vi "dl950_wave_20240517.vi"() -> ()   [LabVIEW 2019]
uses:
  84875dfb-7841-4e1b-95d2-ad8c7a5fa926.vi
  <vilib>/DAQmx/write.llb/DAQmx Write (Analog 1D Wfm NChan NSamp).vi
  <vilib>/DAQmx/create/channels.llb/DAQmx Create Channel (AO-Voltage-Basic).vi
  <vilib>/DAQmx/configure/timing.llb/DAQmx Timing (Sample Clock).vi
  <vilib>/DAQmx/miscellaneous.llb/DAQmx Fill In Error Info.vi
  <instrlib>/Yokogawa DL950 Series/Yokogawa DL950 Series.lvlib
  <resource>/objmgr/daqmx.rc
  <vilib>/measure/NI_MABase.lvlib
panel:
  in  "items":i32[](array[ring]) items=["Peak to Peak", "Amplitude", "Max", "Min", "High", "Low", "Average", "Middle", "Rms", "Standard Deviation", "+Overshoot", "-Overshoot", "Rise", "Fall", "Frequency", "Period", "+Width", "-Width", "Duty Cycle", "Pulse Count", "Burst1 Width", "Burst2 Width", "Average Frequency", "Average Period", "Int1TY", "Int2TY"]
  in  "enable":bool[](array[boolean])
  in  "stop 2":bool
  in  "Tab Control":enum32{"NI AO", "DL950", "load file"}(tab)
  in  "AO Stop":bool
  in  "AO Start":bool
  in  "Physical Channel(s)":tag="cDAQ1Mod1/ao0"
  in  "Min Voltage":dbl=-5.0
  in  "Max Voltage":dbl=5.0
  in  "Sample Clock Source":tag="OnboardClock"
  in  "Sample Rate":dbl=1000.0
  in  "Number of Samples":i32=100
  in  "Output Array":T1(array[cluster])=[{"Waveform Type"=2, "Amplitude"=1.0, "Frequency"=100.0}] {"Frequency" format="%0.2p"; "Amplitude" format="%0.2p"; "Waveform Type" items=["Sine Wave", "Triangle Wave", "Square Wave", "Sawtooth Wave"]}
  in  "offset":dbl=1.0 format="%#_13g"
  in  "square wave duty cycle (%)":dbl=50.0 format="%0.2f"
  out "Waveform Graph 2":waveform(dbl)[](graph)=[{"t0"=timestamp(0 s since 1904-01-01), "dt"=0.001, "Y"=[]}]
  in  "Sample Mode":i32(ring)=10178 items=["Finite Samples", "Continuous Samples", "Hardware Timed Single Point"]
  in  "DAQ Simulation":bool
  out "data":T2
  out "Name of Items":string[](array[string])
  out "Items":dbl[](array[numeric])
  in  "Item Measure":bool
  in  "Item Measure":bool
  in  "Set Apply":bool
  in  "Normal":bool
  in  "open":dbl
  in  "short":dbl
  in  "Open":bool
  in  "Short":bool
  out "Waveform Graph":waveform(dbl)(graph)
  in  "Timeout (10000 ms)":u32=10000
  in  "Sub Channel (0: None)":i16(ring) items=["None", "SCH1", "SCH2", "SCH3", "SCH4", "SCH5", "SCH6", "SCH7", "SCH8", "SCH9", "SCH10", "SCH11", "SCH12", "SCH13", "SCH14", "SCH15", "SCH16", "SCH17", "SCH18", "SCH19", "SCH20", "SCH21", "SCH22", "SCH23", "SCH24", "SCH25", "SCH26", "SCH27", "SCH28", "SCH29", "SCH30", "SCH31", "SCH32", "SCH33", "SCH34", "SCH35", "SCH36", "SCH37", "SCH38", "SCH39", "SCH40", "SCH41", "SCH42", "SCH43", "SCH44", "SCH45", "SCH46", "SCH47", "SCH48", "SCH49", "SCH50", "SCH51", "SCH52", "SCH53", "SCH54", "SCH55", "SCH56", "SCH57", "SCH58", "SCH59", "SCH60", "SCH61", "SCH62", "SCH63", "SCH64"]
  in  "Source (1: CH1)":u16(ring)=1 items=["", "CH1", "CH2", "CH3", "CH4", "CH5", "CH6", "CH7", "CH8", "CH9", "CH10", "CH11", "CH12", "CH13", "CH14", "CH15", "CH16", "MATH1", "MATH2", "MATH3", "MATH4", "MATH5", "MATH6", "MATH7", "MATH8", "EVENT"]
  in  "VISA resource name":refnum<visa-resource-name>="TCPIP0::192.168.0.100::inst0::INSTR"
  in  "Connect":bool
  in  "disconnect":bool
  in  "start":bool
  in  "stop":bool
  in  "freerun":bool
  in  "aquisition":bool
  in  "String":string=":TRIG:SOUT:TYPE ACQ;"
  in  "aquisition STOP":bool
  in  "Vertical Coupling (1: DC)":i32(ring)=1 items=["AC", "DC", "Ground", "AC-RMS", "DC-RMS"]
  in  "Vertical Division (20: 50)":i32(ring)=20 items=["0.1m", "0.2m", "0.5m", "1m", "2m", "5m", "10m", "20m", "50m", "100m", "200m", "500m", "1", "2", "4", "5", "8", "10", "20", "40", "50", "80", "100", "200", "400", "500", "800", "1k", "2k", "4k", "5k", "8k", "10k", "20k", "25k", "50k", "100k", "250k", "500k", "1000k"]
  in  "Time Division (12: 1ms)":i32(ring)=12 items=["100ns", "200ns", "500ns", "1us", "2us", "5us", "10us", "20us", "50us", "100us", "200us", "500us", "1ms", "2ms", "5ms", "10ms", "20ms", "50ms", "100ms", "200ms", "500ms", "1s", "2s", "3s", "4s", "5s", "6s", "10s", "20s", "30s", "1min", "2min", "3min", "4min", "5min", "6min", "10min", "12min", "30min", "1hour", "2hour", "3hour", "4hour", "5hour", "6hour", "8hour", "10hour", "12hour", "1day", "2day", "3day", "4day", "5day"]
  out "Array":dbl[](array[numeric])
  in  "Record Length (0: 10k)":i32(ring) items=["10k", "25k", "50k", "100k", "250k", "500k", "1M", "2.5M", "5M", "10M", "25M", "50M", "100M", "250M", "500M", "1G", "2G", "4G", "5G", "10G", "20G", "50G"]
  in  "Acquisition Mode (0: Normal)":i32(ring) items=["Normal", "Average", "Envelope"]
  in  "inpuPara":T3={"Rising[%] 1"=63.0, "Rising[%] 2"=99.0, "Falling[%]"=37.0}
  out "calculation":u32
  out "itemMeasure":u32
  out "Oscilloscope":u32
  out "Loop":u32
  in  "End Point(1000)":i64=1000
  in  "Record Number (0)":i32
  in  "Start Point(0)":i64
  out "task out":refnum<k21>
  out "SampQuant.SampPerChan":dbl
  out "SampClk.Rate":dbl
  in  "Channel (1: CH1)":u16(ring)=1 items=["", "CH1", "CH2", "CH3", "CH4", "CH5", "CH6", "CH7", "CH8", "CH9", "CH10", "CH11", "CH12", "CH13", "CH14", "CH15", "CH16", "RMATH1", "RMATH2", "RMATH3", "RMATH4", "RMATH5", "RMATH6", "RMATH7", "RMATH8", "RMATH9", "RMATH10", "RMATH11", "RMATH12", "RMATH13", "RMATH14", "RMATH15", "RMATH16"]
  in  "sub Channel (1: CH1)":u16(ring)=1 items=["", "CH1", "CH2", "CH3", "CH4", "CH5", "CH6", "CH7", "CH8", "CH9", "CH10", "CH11", "CH12", "CH13", "CH14", "CH15", "CH16", "RMATH1", "RMATH2", "RMATH3", "RMATH4", "RMATH5", "RMATH6", "RMATH7", "RMATH8", "RMATH9", "RMATH10", "RMATH11", "RMATH12", "RMATH13", "RMATH14", "RMATH15", "RMATH16"]
  in  "Enable Channel (True)":bool=TRUE
  in  "Reset":bool
  in  "write":bool
  out "read buffer":string
  in  "String 2":string=":FILE:SAVE?;"
  in  "Numeric":u32=20
  in  "response":bool
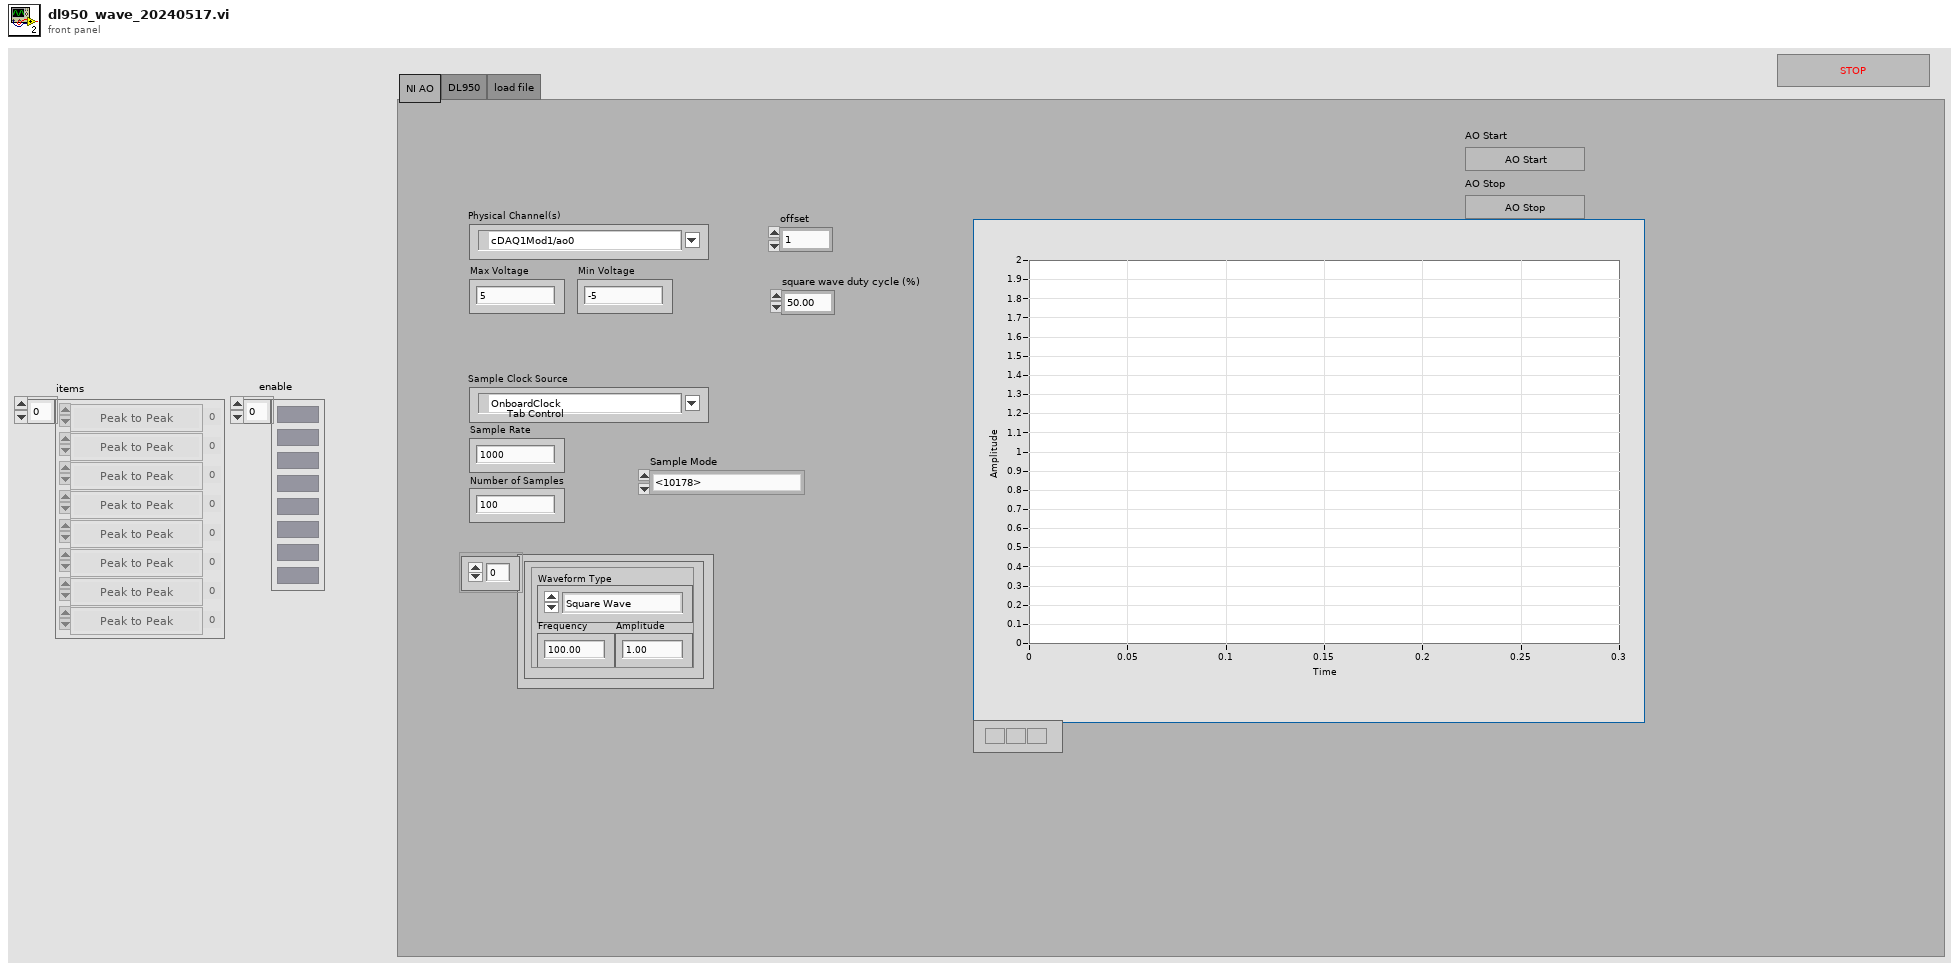
[diagram p1: front panel]
types:
  T1 = cluster{"Waveform Type":u16, "Amplitude":dbl, "Frequency":dbl}[]
  T2 = cluster{"pulse":i32, "Rising[%] 1":dbl, "Rising[%] 2":dbl, "Falling[%]":dbl, "R_max":dbl}
  T3 = cluster{"Rising[%] 1":dbl, "Rising[%] 2":dbl, "Falling[%]":dbl}
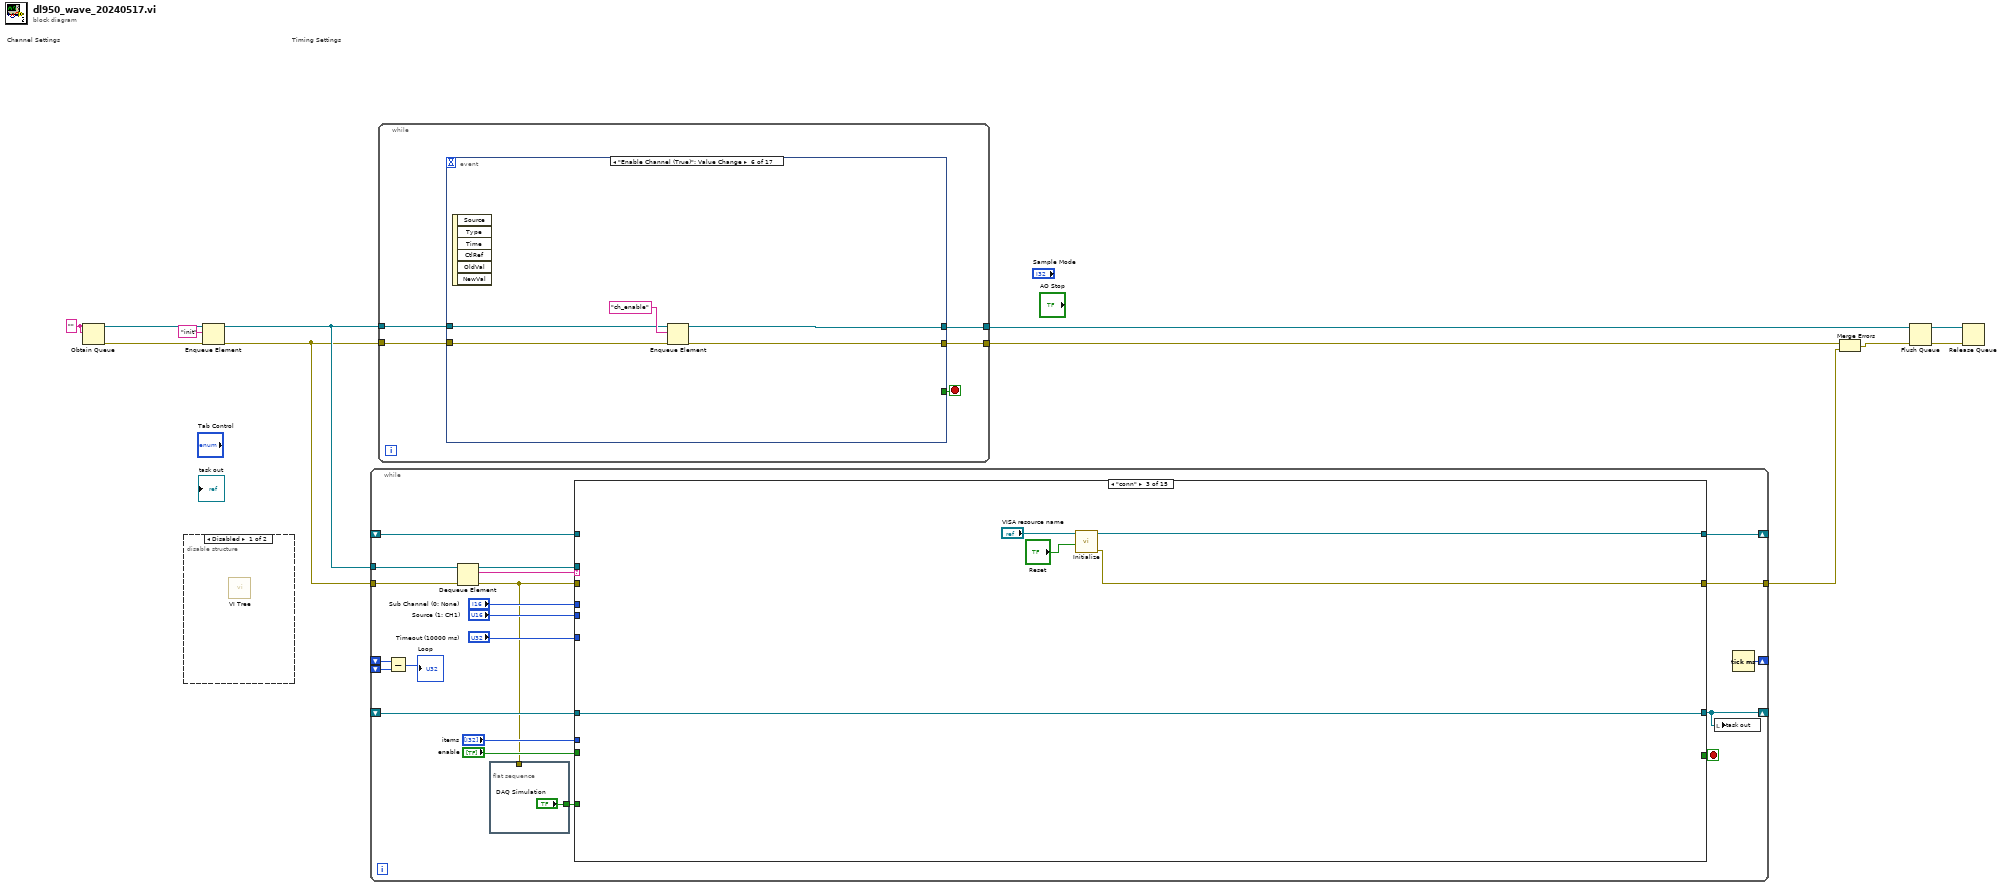
[diagram p0: block diagram]
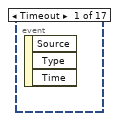
[diagram p3: hidden frame]
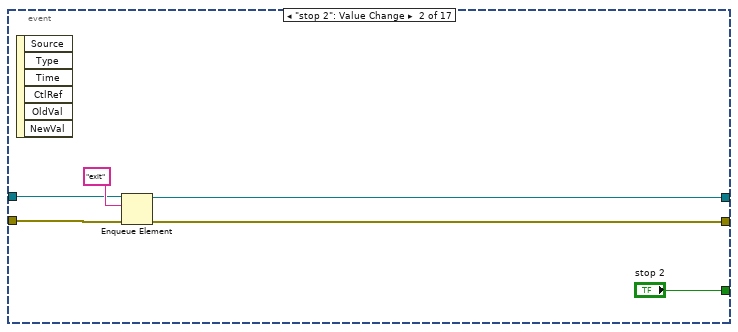
[diagram p4: hidden frame]
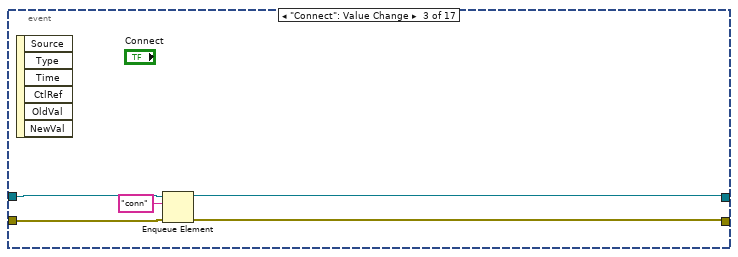
[diagram p5: hidden frame]
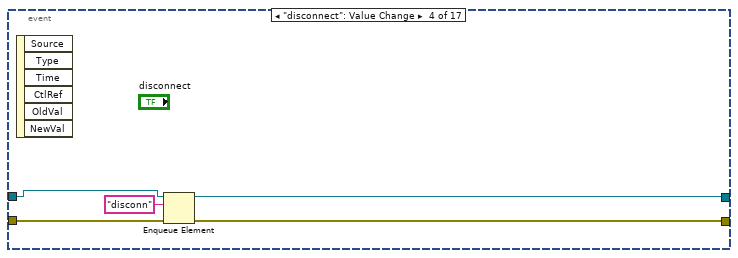
[diagram p6: hidden frame]
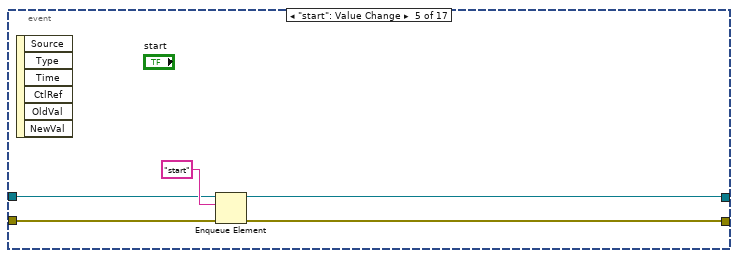
[diagram p7: hidden frame]
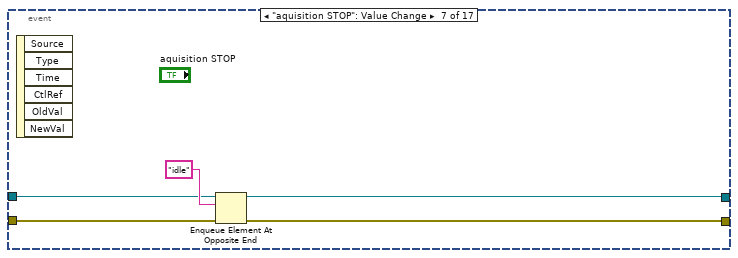
[diagram p8: hidden frame]
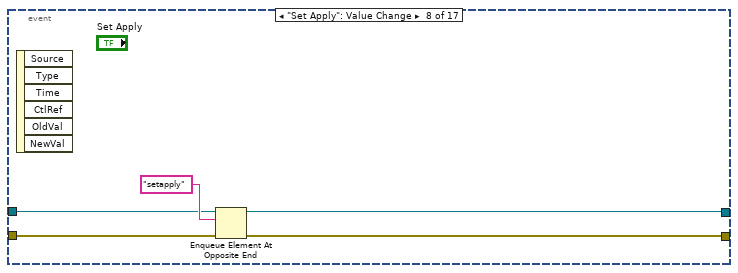
[diagram p9: hidden frame]
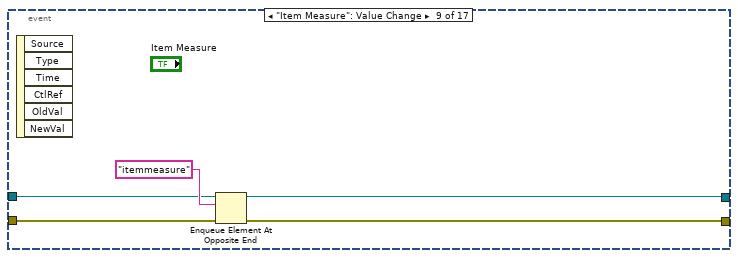
[diagram p10: hidden frame]
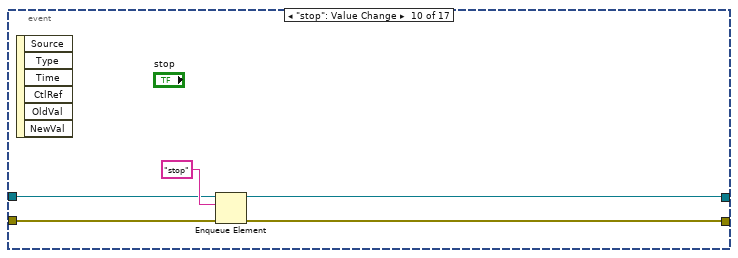
[diagram p11: hidden frame]
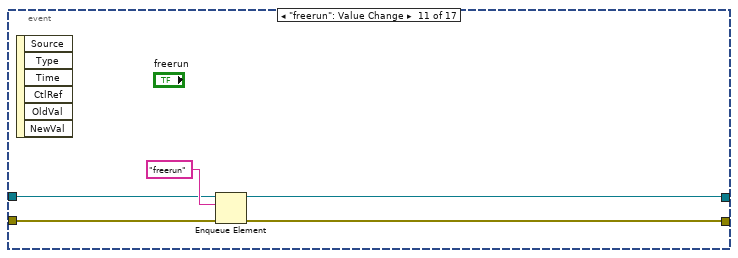
[diagram p12: hidden frame]
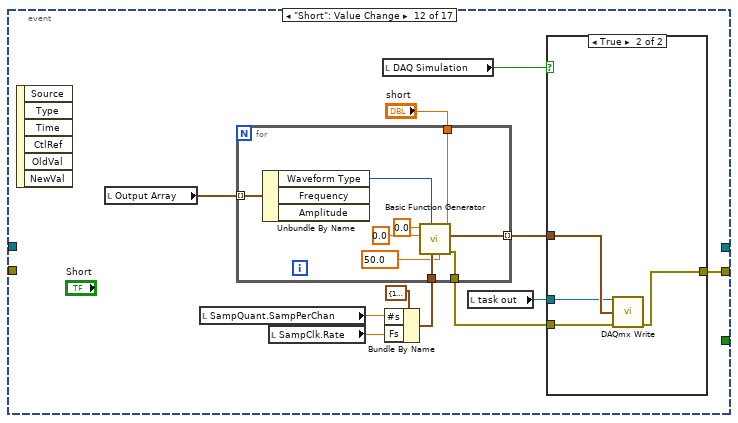
[diagram p13: hidden frame]
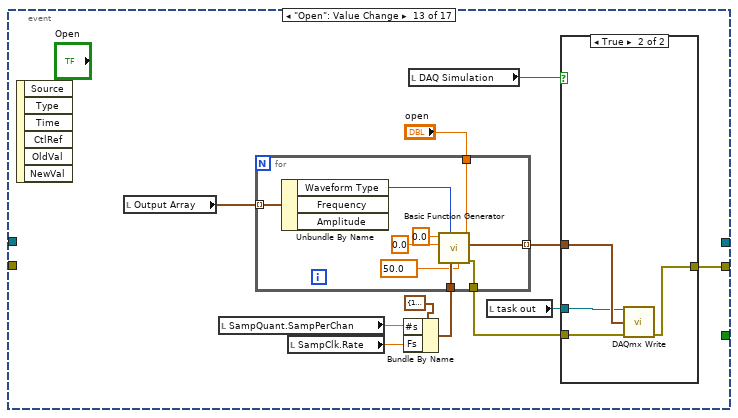
[diagram p15: hidden frame]
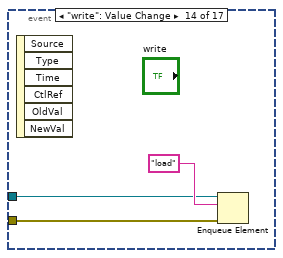
[diagram p17: hidden frame]
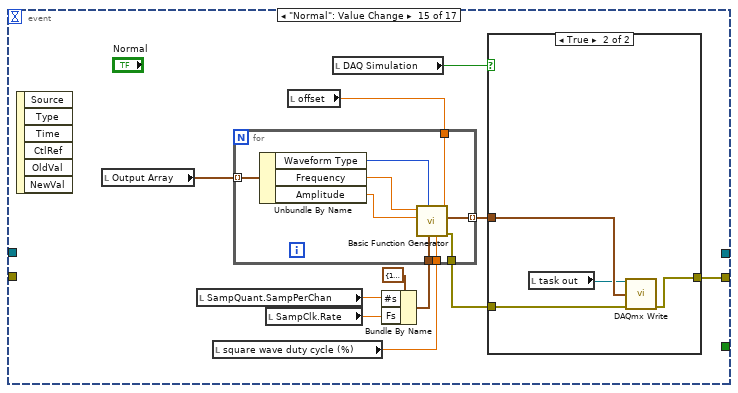
[diagram p18: hidden frame]
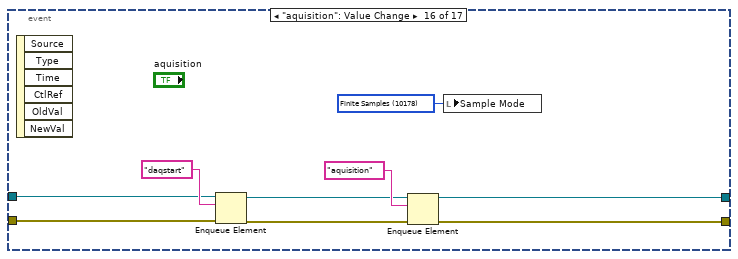
[diagram p20: hidden frame]
diagram:
  w1 = "" ("name (unnamed)")
  # "Timing Settings"
  # "Channel Settings"
  n1 = Obtain Queue(name (unnamed)=w1, element data type=w1) -> (queue out=w12:refnum<queue>, error out=w11:errorcluster)  [unwired: 3 in, 1 out]
  n2 = disable-structure shown="Disabled" {
    frame Disabled {
      n3 = call <instrlib>:"VI Tree.vi"() -> ()  [unwired: 12 in]
    }
    frame Enabled {
    }
  }
  n4 = Enqueue Element(queue=w12, element="init", error in (no error)=w11) -> (queue out=w9:refnum<queue>, error out=w8:errorcluster)  [unwired: 1 in, 1 out]
  n5 = while {
    tunnel: w9 -> [w33]
    tunnel: w8 -> [w32]
    tunnel: [w29] -> w6
    shift-right: [w28] -> _
    shift-left: _ -> [w27]
    shift-right: [w22] -> _
    shift-left: _ -> [w21]
    shift-left: _ -> [w20]
    shift-right: [w17] -> _
    shift-left: _ -> [w18]
    stop <- w30 stop-if-true
    n6 = Subtract(x=w21, y=w20) -> (x-y=→"Loop":u32)
    n7 = Dequeue Element(queue=w33, error in (no error)=w32) -> (queue out=w23:refnum<queue>, element=w31:string, error out=w14:errorcluster)  [unwired: 1 in, 1 out]
    n8 = flat-sequence {
      tunnel: w14 -> [_]
      tunnel: ["DAQ Simulation"] -> w13
      frame #0 {
      }
    }
    n9 = case shown="\"conn\"" w31 {
      tunnel: [_ TRUE _ _ _ _ _ _ _ _ _ _ _ _ _] -> w30
      tunnel: [w36 w40 w42 w50 w80 w96 w99 w106 w112 w122 w210 w238 w284 w295 w301] -> w29
      tunnel: w14 -> [w36 w40 _ w52 w64 w97 w100 w107 w113 w148 w211 _ w290 w296 w302]
      tunnel: [w37 w39 w43 w51 w81 w95 w101 w108 w114 w134 w212 w239 w292 w298 w305] -> w28
      tunnel: w27 -> [w37 w39 _ w53 w65 w95 w102 w109 w115 w146 w213 w239 w292 w298 w305]
      tunnel: "Source (1: CH1)" -> [_ _ _ _ w63 _ _ _ _ w132 w207 _ _ _ _]
      tunnel: "Sub Channel (0: None)" -> [_ _ _ _ w79 _ _ _ _ w131 w206 _ _ _ _]
      tunnel: "Timeout (10000 ms)" -> [_ _ _ _ _ _ _ _ _ w153 _ _ _ _ _]
      tunnel: w23 -> [_ _ _ _ _ _ _ _ _ w149 _ _ w289 w297 _]
      tunnel: [w35 w38 w45 w54 w83 w94 w98 w104 w110 w140 w214 w237 w285 w294 w307] -> w17
      tunnel: w18 -> [w35 w38 w45 w54 w83 w94 w98 w104 w110 w141 w214 _ w286 w294 w307]
      tunnel: "items" -> [_ _ _ _ w78 _ _ _ _ w130 w209 _ _ _ _]
      tunnel: "enable" -> [_ _ _ _ w77 _ _ _ _ w129 w208 _ _ _ _]
      tunnel: w13 -> [_ _ _ _ _ _ _ _ _ w116 _ w236 _ w293 _]
      frame "False", Default {
      }
      frame "exit" {
      }
      frame "conn" {
        n10 = call <instrlib>:"Initialize.vi"("Reset (True)"="Reset", "VISA resource name"="VISA resource name") -> ("error out"=w42:errorcluster, "VISA resource name out"=w43:refnum<visa-resource-name>)  [unwired: 8 in]
      }
      frame "ch_enable" {
        n11 = call <instrlib>:"Configure Channel.vi"("VISA resource name"=w53, "Channel (1: CH1)"="Channel (1: CH1)", "Enable Channel (True)"="Enable Channel (True)", "sub Channel (1: CH1)"="sub Channel (1: CH1)", "error in (no error)"=w52) -> ("VISA resource name out"=w51:refnum<visa-resource-name>, "error out"=w50:errorcluster)  [unwired: 9 in]
      }
      frame "setapply" {
        n12 = Format Into String ("文字列にフォーマット")(format string="CHAN%d:", w63) -> (resulting string=w72:string)  [unwired: 2 in, 1 out]
        n13 = Pick Line ("ライン選択")(string ("")=w72, multi-line string="COUP AC;\nCOUP DC;\nCOUP GND;\nCOUP ACRMS;\nCOUP DCRMS;", line index="Vertical Coupling (1: DC)") -> (output string=w73:string)
        n14 = call <instrlib>:"Configure Acquisition.vi"("VISA resource name"=w65, "Record Length (0: 10k)"="Record Length (0: 10k)", "Acquisition Mode (0: Normal)"="Acquisition Mode (0: Normal)", "error in (no error)"=w64) -> ("VISA resource name out"=w60:refnum<visa-resource-name>, "error out"=w58:errorcluster)  [unwired: 10 in]
        n15 = call <instrlib>:"Configure Timebase.vi"("VISA resource name"=w60, "Time Division (12: 1ms)"="Time Division (12: 1ms)", "error in (no error)"=w58) -> ("VISA resource name out"=w59:refnum<visa-resource-name>, "error out"=w57:errorcluster)  [unwired: 11 in]
        n16 = Pick Line ("ライン選択")(string ("")=w73, multi-line string="VDIV 0.0001;\nVDIV 0.0002;\nVDIV 0.0005;\nVDIV 0.001;\nVDIV 0.002;\nVDIV 0.005;\nVDIV 0.01;\nVDIV 0.02;\nVDIV 0.05;\nVDIV 0.1;\nVDIV 0.2;\nVDIV 0.5;\nVDIV 1;\nVDIV 2;\nVDIV 4;\nVDIV 5;\nVDIV 8;\nVDIV 10;\nVDIV 20;\nVDIV 40;\nVDIV 50;\nVDIV 80;\nVDIV 100;\nVDIV 200;\nVDIV 400;\nVDIV 500;\nVDIV 800;\nVDIV 1000;\nVDIV 2000;\nVDIV 4000;\nVDIV 5000;\nVDIV 8000;\nVDIV 10000;\nVDIV 20000;\nVDIV 25000;\nVDIV 50000;\nVDIV 100000;\nVDIV 250000;\nVDIV 500000;\nVDIV 1000000;", line index="Vertical Division (20: 50)") -> (output string=w68:string)
        n17 = VISA Write ("VISA書き込み")(VISA resource name=w59, write buffer=w68, error in (no error)=w57) -> (VISA resource name out=w56:refnum<visa-resource-name>, error out=w55:errorcluster)  [unwired: 1 out]
        n18 = property on="Measurement Item (0: Peak to Peak)" class="Ring (strict)"(error in=w55) -> (error out=w76:errorcluster, "Strings []"=w75:string[])  [unwired: 1 in, 1 out]
        n19 = for {
          tunnel: w79 -> [w85]
          tunnel: w63 -> [w84]
          shift-right: [w92] -> w81
          shift-left: w56 -> [w93]
          shift-right: [w90] -> w80
          shift-left: w76 -> [w91]
          tunnel: w77 -> [w86] mode=indexing
          tunnel: w78 -> [w88] mode=indexing
          tunnel: w75 -> [w89]
          tunnel: [w87] -> w74 mode=indexing if=w86
          n20 = call <instrlib>:"Configure Measurement Item.vi"("VISA resource name"=w93, "Source (1: CH1)"=w84, "Sub Channel (0: None)"=w85, "Measurement Item (0: Peak to Peak)"=w88, "Enable Measurement Item (False)"=w86, "error in (no error)"=w91) -> ("VISA resource name out"=w92:refnum<visa-resource-name>, "error out"=w90:errorcluster)  [unwired: 8 in]
          n21 = Index Array(array=w89, index=w88) -> (element=w87:string)
        }
        "Name of Items" <- w74
      }
      frame "disconn" {
        n22 = call <instrlib>:"Close.vi"("error in (no error)"=w97, "VISA resource name"=w95) -> ("error out"=w96:errorcluster)  [unwired: 9 in]
      }
      frame "start" {
        w103 = ":STAR;"  # Initiate
        n23 = VISA Write ("VISA書き込み")(VISA resource name=w102, write buffer=w103, error in (no error)=w100) -> (VISA resource name out=w101:refnum<visa-resource-name>, error out=w99:errorcluster)  [unwired: 1 out]
      }
      frame "stop" {
        n24 = VISA Write ("VISA書き込み")(VISA resource name=w109, write buffer=":STOP;", error in (no error)=w107) -> (VISA resource name out=w108:refnum<visa-resource-name>, error out=w106:errorcluster)  [unwired: 1 out]
      }
      frame "freerun" {
        n25 = VISA Write ("VISA書き込み")(VISA resource name=w115, write buffer="String", error in (no error)=w113) -> (VISA resource name out=w114:refnum<visa-resource-name>, error out=w112:errorcluster)  [unwired: 1 out]
      }
      frame "aquisition" {
        w147 = ":STAR;"  # Initiate
        n26 = Enqueue Element(queue=w149, element="aquisition", error in (no error)=w148) -> (error out=w145:errorcluster)  [unwired: 1 in, 2 out]
        n27 = VISA Write ("VISA書き込み")(VISA resource name=w146, write buffer=w147, error in (no error)=w145) -> (VISA resource name out=w143:refnum<visa-resource-name>, error out=w139:errorcluster)  [unwired: 1 out]
        n28 = call "Stall Data Flow.vim"("value in"=w139, "milliseconds to wait"=u32 200) -> ("value out"=w137:errorcluster)  [unwired: 1 out]
        n29 = case shown="True" w116 {
          tunnel: w141 -> [w156 w160]
          tunnel: [w156 w159] -> w140
          tunnel: w137 -> [w155 w158]
          tunnel: [w155 w157] -> w136
          frame False {
          }
          frame True {
            n30 = call <vilib>:"DAQmx Start Task.vi"("task/channels in"=w160, "error in"=w158) -> ("task out"=w163:refnum<k21>, "error out"=w162:errorcluster)  [unwired: 12 in]
            n31 = call <vilib>:"DAQmx Wait Until Done.vi"("task/channels in"=w163, "error in"=w162) -> ("task out"=w161:refnum<k21>, "error out"=w157:errorcluster)  [unwired: 12 in]
            n32 = call <vilib>:"DAQmx Stop Task.vi"("task/channels in"=w161, "error in"=w157) -> ("task out"=w159:refnum<k21>)  [unwired: 12 in, 1 out]
          }
        }
        n33 = VISA Write ("VISA書き込み")(VISA resource name=w143, write buffer=":STOP;", error in (no error)=w136) -> (VISA resource name out=w142:refnum<visa-resource-name>, error out=w121:errorcluster)  [unwired: 1 out]
        n34 = flat-sequence {
          tunnel: w121 -> [w165]
          tunnel: [w165] -> w120
          tunnel: [w164] -> w117
          frame #0 {
            n35 = Tick Count (ms)() -> (millisecond timer value=w164:u32)
          }
        }
        n36 = call "waveAquis.vi"("Timeout (10000 ms)"=w153, "Sub Channel(0: None)"=w131, "End Point(1000)"=i64 -1, "Source (1: CH1)"=w132, "error in (no error)"=w120, "Start Point(0)"="Start Point(0)", "Record Number (0)"="Record Number (0)", "VISA resource name"=w142) -> ("error out"=w125:errorcluster, "Waveform Data"=w128:waveform(dbl), "VISA resource name out"=w135:refnum<visa-resource-name>)  [unwired: 1 in]
        "Waveform Graph" <- w128
        n37 = flat-sequence {
          tunnel: w125 -> [w173]
          tunnel: [w173] -> w124
          tunnel: [w172] -> w118
          frame #0 {
            n38 = Tick Count (ms)() -> (millisecond timer value=w172:u32)
          }
        }
        n39 = case shown="True" "Item Measure" {
          tunnel: w135 -> [w175 w184]
          tunnel: [w175 w183] -> w134
          tunnel: w125 -> [w174 w182]
          tunnel: [w174 w181] -> w122
          tunnel: w132 -> [_ w180]
          tunnel: w131 -> [_ w179]
          tunnel: w130 -> [_ w178]
          tunnel: w129 -> [_ w177]
          frame False {
          }
          frame True {
            n40 = for {
              tunnel: w184 -> [w193]
              tunnel: [w192] -> w183
              tunnel: w182 -> [w191]
              tunnel: [w190] -> w181
              tunnel: w178 -> [w189] mode=indexing
              tunnel: w177 -> [w188] mode=indexing
              tunnel: w180 -> [w187]
              tunnel: w179 -> [w186]
              tunnel: [w185] -> w176 mode=indexing
              n41 = case shown="True" w188 {
                tunnel: w193 -> [w196 w204]
                tunnel: [w196 w203] -> w192
                tunnel: w191 -> [w195 w202]
                tunnel: [w195 w201] -> w190
                tunnel: w189 -> [_ w200]
                tunnel: w187 -> [_ w199]
                tunnel: w186 -> [_ w198]
                tunnel: [0.0 ("Measurement Value") w197] -> w185
                frame False {
                }
                frame True {
                  n42 = call <instrlib>:"Read Waveform Measurement.vi"("VISA resource name"=w204, "Source (1: CH1)"=w199, "Sub Channel (0: None)"=w198, "Measurement Item (0: Peak to Peak)"=w200, "error in (no error)"=w202) -> ("VISA resource name out"=w203:refnum<visa-resource-name>, "Measurement Value"=w197:dbl, "error out"=w201:errorcluster)  [unwired: 8 in]
                }
              }
            }
            "Items" <- w176
          }
        }
        n43 = Subtract(x=w118, y=w117) -> (x-y=→"Oscilloscope":u32)
        n44 = call "signalAnalysis.vi"("error in (no error)"=w124, "inpuPara"="inpuPara", "data_scope"=w128) -> ("error out"=w123:errorcluster, "data"=→"data":T2)  [unwired: 7 in]
        n45 = flat-sequence {
          tunnel: w123 -> [_]
          tunnel: w118 -> [w170]
          frame #0 {
            n46 = Tick Count (ms)() -> (millisecond timer value=w171:u32)
            n47 = Subtract(x=w171, y=w170) -> (x-y=→"calculation":u32)
          }
        }
        n48 = flat-sequence {
          tunnel: w118 -> [w167]
          tunnel: w122 -> [_]
          frame #0 {
            n49 = Tick Count (ms)() -> (millisecond timer value=w168:u32)
            n50 = Subtract(x=w168, y=w167) -> (x-y=→"itemMeasure":u32)
          }
        }
      }
      frame "itemmeasure" {
        n51 = for {
          tunnel: w213 -> [w223]
          tunnel: [w222] -> w212
          tunnel: w211 -> [w221]
          tunnel: [w220] -> w210
          tunnel: w209 -> [w219] mode=indexing
          tunnel: w208 -> [w218] mode=indexing
          tunnel: w207 -> [w217]
          tunnel: w206 -> [w216]
          tunnel: [w215] -> w205 mode=indexing
          n52 = case shown="True" w218 {
            tunnel: w223 -> [w226 w234]
            tunnel: [w226 w233] -> w222
            tunnel: w221 -> [w225 w232]
            tunnel: [w225 w231] -> w220
            tunnel: w219 -> [_ w230]
            tunnel: w217 -> [_ w229]
            tunnel: w216 -> [_ w228]
            tunnel: [0.0 ("Measurement Value") w227] -> w215
            frame False {
            }
            frame True {
              n53 = call <instrlib>:"Read Waveform Measurement.vi"("VISA resource name"=w234, "Source (1: CH1)"=w229, "Sub Channel (0: None)"=w228, "Measurement Item (0: Peak to Peak)"=w230, "error in (no error)"=w232) -> ("VISA resource name out"=w233:refnum<visa-resource-name>, "Measurement Value"=w227:dbl, "error out"=w231:errorcluster)  [unwired: 8 in]
            }
          }
        }
        "Array" <- w205
      }
      frame "daqstart" {
        n54 = local read "Sample Mode"() -> (w235:i32)
        n55 = case shown="True" w236 {
          tunnel: [_ w243] -> w238
          tunnel: [refnum<k21> refnum ("task out") w242] -> w237
          tunnel: w235 -> [_ w241]
          frame False {
          }
          frame True {
            n56 = stacked-sequence {
              seq-local: [w247 _] -> [_ w265]
              seq-local: [w246 _] -> [_ w263]
              seq-local: [w245 _] -> [_ w264]
              tunnel: [w246 _] -> _
              tunnel: [w245 _] -> _
              tunnel: [w247 _] -> _
              tunnel: [w248 _] -> w243
              tunnel: [_ w261] -> w242
              tunnel: w241 -> [w244 w262]
              frame #0 {
                n57 = call-poly <vilib>:"DAQmx Create Virtual Channel.vi"("maximum value"="Max Voltage", "minimum value"="Min Voltage", "physical channels"="Physical Channel(s)") -> ("task out"=w255:refnum<k21>, "error out"=w256:errorcluster)  [unwired: 11 in]
                n58 = call-poly <vilib>:"DAQmx Timing.vi"("task/channels in"=w255, "sample mode"=w244, "samples per channel"="Number of Samples", "rate"="Sample Rate", "source"="Sample Clock Source", "error in"=w256) -> ("task out"=w258:refnum<k21>, "error out"=w257:errorcluster)  [unwired: 8 in]
                n59 = property class="DAQmx Timing"(reference=w258, error in=w257) -> (reference out=w247:refnum<k21>, error out=w248:errorcluster, "SampQuant.SampPerChan"=w246:dbl, "SampClk.Rate"=w245:dbl)
                "SampQuant.SampPerChan" <- w246
                "SampClk.Rate" <- w245
              }
              frame #1 {
                n60 = Bundle By Name(cluster=cluster{"Fs":dbl, "#s":dbl} {"Fs"=1000.0, "#s"=1000.0} ("sampling info"), "#s"=w263, "Fs"=w264) -> (w267:cluster{"Fs":dbl, "#s":dbl})
                n61 = for {
                  tunnel: w267 -> [w283]
                  tunnel: [w282] -> w268
                  tunnel: "Output Array" -> [w281] mode=indexing
                  tunnel: [w277] -> w270 mode=indexing
                  n62 = Unbundle By Name(w281) -> ("Waveform Type"=w280:u16, "Frequency"=w279:dbl, "Amplitude"=w278:dbl)
                  n63 = call <vilib>:"Basic Function Generator.vi"("offset"="offset", "square wave duty cycle (%)"="square wave duty cycle (%)", "sampling info"=w283, "signal type"=w280, "amplitude"=w278, "frequency"=w279) -> ("error out"=w282:errorcluster, "signal out"=w277:waveform(dbl))  [unwired: 3 in, 1 out]
                }
                "Waveform Graph 2" <- w270
                n64 = call-poly <vilib>:"DAQmx Write.vi"("task/channels in"=w265, "data"=w270, "error in"=w268) -> ("task out"=w260:refnum<k21>, "error out"=w259:errorcluster)  [unwired: 10 in, 1 out]
                n65 = case shown="1" w262 {
                  tunnel: [w271 w273] -> w261
                  tunnel: w260 -> [w271 w274]
                  tunnel: w259 -> [_ w272]
                  frame 0, Default {
                  }
                  frame 1 {
                    n66 = call <vilib>:"DAQmx Start Task.vi"("task/channels in"=w274, "error in"=w272) -> ("task out"=w273:refnum<k21>)  [unwired: 12 in, 1 out]
                  }
                }
              }
            }
          }
        }
      }
      frame "aostart" {
        n67 = Enqueue Element(queue=w289, element="aostart", error in (no error)=w290) -> (error out=w287:errorcluster)  [unwired: 1 in, 2 out]
        n68 = call <vilib>:"DAQmx Is Task Done.vi"("task/channels in"=w286, "error in"=w287) -> ("task out"=w285:refnum<k21>, "error out"=w284:errorcluster)  [unwired: 11 in, 1 out]
        n69 = Wait Until Next ms Multiple(millisecond multiple=u32 100) -> ()  [unwired: 1 out]
      }
      frame "idle" {
        n70 = Flush Queue(queue=w297, error in (no error)=w296) -> (error out=w295:errorcluster)  [unwired: 2 out]
        n71 = case shown="True" w293 {
          tunnel: w294 -> [_ w299]
          frame False {
          }
          frame True {
            n72 = call <vilib>:"DAQmx Clear Task.vi"("task in"=w299) -> ()  [unwired: 14 in, 1 out]
          }
        }
      }
      frame "load" {
        n73 = VISA Write ("VISA書き込み")(VISA resource name=w305, write buffer="String 2", error in (no error)=w302) -> (VISA resource name out=w304:refnum<visa-resource-name>, error out=w303:errorcluster)  [unwired: 1 out]
        n74 = case shown="True" "response" {
          tunnel: w304 -> [_ w312]
          tunnel: w303 -> [w308 w311]
          tunnel: [w308 w310] -> w301
          frame False {
          }
          frame True {
            n75 = VISA Read ("VISA読み取り")(VISA resource name=w312, byte count="Numeric", error in (no error)=w311) -> (read buffer=→"read buffer":string, error out=w310:errorcluster)  [unwired: 2 out]
          }
        }
      }
    }
    n76 = local write "task out"(w17) -> ()
    n77 = Tick Count (ms)() -> (millisecond timer value=w22:u32)
  }
  n78 = while {
    tunnel: w9 -> [w317]
    tunnel: w8 -> [w316]
    tunnel: [w315] -> w5
    tunnel: [w314] -> w7
    stop <- w318 stop-if-true
    n79 = event shown="[5] \"Enable Channel (True)\": Value Change" {
      selector: _ -> [_ _ _ _ _ _ _ _ _ _ _ _ _ _ _ _ _]
      dyn-events: _ -> [_ _ _ _ _ _ _ _ _ _ _ _ _ _ _ _ _]
      timeout: _ -> [_ _ _ _ _ _ _ _ _ _ _ _ _ _ _ _ _]
      tunnel: [_ "stop 2" _ _ _ _ _ _ _ _ _ _ _ _ _ _ _] -> w318
      tunnel: w317 -> [_ w322 w328 w333 w338 w343 w348 w353 w358 w363 w368 _ _ w421 _ w455 w461]
      tunnel: w316 -> [_ w321 w326 w332 w337 w341 w347 w352 w357 w362 w367 _ _ w420 _ w454 w459]
      tunnel: [_ w320 w327 w331 w336 w342 w346 w351 w356 w361 w366 _ _ _ _ w450 w464] -> w315
      tunnel: [_ w319 w325 w330 w335 w340 w345 w350 w355 w360 w365 w371 w397 _ w424 w449 w463] -> w314
      event Timeout {
        n80 = event-data() -> ()  [unwired: 1 in, 3 out]
      }
      event "stop 2": Value Change {
        n81 = event-data() -> ()  [unwired: 1 in, 6 out]
        n82 = Enqueue Element(queue=w322, element="exit", error in (no error)=w321) -> (queue out=w320:refnum<queue>, error out=w319:errorcluster)  [unwired: 1 in, 1 out]
      }
      event "Connect": Value Change {
        n83 = event-data() -> ()  [unwired: 1 in, 6 out]
        n84 = Enqueue Element(queue=w328, element="conn", error in (no error)=w326) -> (queue out=w327:refnum<queue>, error out=w325:errorcluster)  [unwired: 1 in, 1 out]
      }
      event "disconnect": Value Change {
        n85 = event-data() -> ()  [unwired: 1 in, 6 out]
        n86 = Enqueue Element(queue=w333, element="disconn", error in (no error)=w332) -> (queue out=w331:refnum<queue>, error out=w330:errorcluster)  [unwired: 1 in, 1 out]
      }
      event "start": Value Change {
        n87 = event-data() -> ()  [unwired: 1 in, 6 out]
        n88 = Enqueue Element(queue=w338, element="start", error in (no error)=w337) -> (queue out=w336:refnum<queue>, error out=w335:errorcluster)  [unwired: 1 in, 1 out]
      }
      event "Enable Channel (True)": Value Change {
        n89 = event-data() -> ()  [unwired: 1 in, 6 out]
        n90 = Enqueue Element(queue=w343, element="ch_enable", error in (no error)=w341) -> (queue out=w342:refnum<queue>, error out=w340:errorcluster)  [unwired: 1 in, 1 out]
      }
      event "aquisition STOP": Value Change {
        n91 = event-data() -> ()  [unwired: 1 in, 6 out]
        n92 = Enqueue Element At Opposite End(queue=w348, element="idle", error in (no error)=w347) -> (queue out=w346:refnum<queue>, error out=w345:errorcluster)  [unwired: 1 in, 1 out]
      }
      event "Set Apply": Value Change {
        n93 = event-data() -> ()  [unwired: 1 in, 6 out]
        n94 = Enqueue Element At Opposite End(queue=w353, element="setapply", error in (no error)=w352) -> (queue out=w351:refnum<queue>, error out=w350:errorcluster)  [unwired: 1 in, 1 out]
      }
      event "Item Measure": Value Change {
        n95 = event-data() -> ()  [unwired: 1 in, 6 out]
        n96 = Enqueue Element At Opposite End(queue=w358, element="itemmeasure", error in (no error)=w357) -> (queue out=w356:refnum<queue>, error out=w355:errorcluster)  [unwired: 1 in, 1 out]
      }
      event "stop": Value Change {
        n97 = event-data() -> ()  [unwired: 1 in, 6 out]
        n98 = Enqueue Element(queue=w363, element="stop", error in (no error)=w362) -> (queue out=w361:refnum<queue>, error out=w360:errorcluster)  [unwired: 1 in, 1 out]
      }
      event "freerun": Value Change {
        n99 = event-data() -> ()  [unwired: 1 in, 6 out]
        n100 = Enqueue Element(queue=w368, element="freerun", error in (no error)=w367) -> (queue out=w366:refnum<queue>, error out=w365:errorcluster)  [unwired: 1 in, 1 out]
      }
      event "Short": Value Change {
        n101 = event-data() -> ()  [unwired: 1 in, 6 out]
        n102 = local read "Output Array"() -> (w376:T1)
        n103 = local read "SampQuant.SampPerChan"() -> (w374:dbl)
        n104 = local read "SampClk.Rate"() -> (w373:dbl)
        n105 = local read "DAQ Simulation"() -> (w370:bool)
        n106 = Bundle By Name(cluster=cluster{"Fs":dbl, "#s":dbl} {"Fs"=1000.0, "#s"=1000.0} ("sampling info"), "#s"=w374, "Fs"=w373) -> (w380:cluster{"Fs":dbl, "#s":dbl})
        n107 = for {
          tunnel: w380 -> [w394]
          tunnel: [w393] -> w379
          tunnel: [w392] -> w378 mode=indexing
          tunnel: w376 -> [w390] mode=indexing
          tunnel: "short" -> [w386]
          n108 = Unbundle By Name(w390) -> ("Waveform Type"=w389:u16)  [unwired: 2 out]
          n109 = call <vilib>:"Basic Function Generator.vi"("offset"=w386, "square wave duty cycle (%)"=50.0 ("square wave duty cycle (%) 2"), "sampling info"=w394, "signal type"=w389, "amplitude"=0.0, "frequency"=0.0) -> ("error out"=w393:errorcluster, "signal out"=w392:waveform(dbl))  [unwired: 3 in, 1 out]
        }
        n110 = local read "task out"() -> (w372:refnum<k21>)
        n111 = case shown="True" w370 {
          tunnel: w379 -> [w381 w385]
          tunnel: w378 -> [_ w384]
          tunnel: w372 -> [_ w383]
          tunnel: [w381 w382] -> w371
          frame False {
          }
          frame True {
            n112 = call-poly <vilib>:"DAQmx Write.vi"("task/channels in"=w383, "data"=w384, "error in"=w385) -> ("error out"=w382:errorcluster)  [unwired: 10 in, 2 out]
          }
        }
      }
      event "Open": Value Change {
        n113 = event-data() -> ()  [unwired: 1 in, 6 out]
        n114 = local read "Output Array"() -> (w402:T1)
        n115 = local read "SampQuant.SampPerChan"() -> (w401:dbl)
        n116 = local read "SampClk.Rate"() -> (w400:dbl)
        n117 = Bundle By Name(cluster=cluster{"Fs":dbl, "#s":dbl} {"Fs"=1000.0, "#s"=1000.0} ("sampling info"), "#s"=w401, "Fs"=w400) -> (w405:cluster{"Fs":dbl, "#s":dbl})
        n118 = for {
          tunnel: w405 -> [w419]
          tunnel: [w418] -> w404
          tunnel: [w417] -> w403 mode=indexing
          tunnel: w402 -> [w415] mode=indexing
          tunnel: "open" -> [w411]
          n119 = Unbundle By Name(w415) -> ("Waveform Type"=w414:u16)  [unwired: 2 out]
          n120 = call <vilib>:"Basic Function Generator.vi"("offset"=w411, "square wave duty cycle (%)"=50.0 ("square wave duty cycle (%) 2"), "sampling info"=w419, "signal type"=w414, "amplitude"=0.0, "frequency"=0.0) -> ("error out"=w418:errorcluster, "signal out"=w417:waveform(dbl))  [unwired: 3 in, 1 out]
        }
        n121 = local read "DAQ Simulation"() -> (w395:bool)
        n122 = local read "task out"() -> (w399:refnum<k21>)
        n123 = case shown="True" w395 {
          tunnel: w404 -> [w406 w410]
          tunnel: w403 -> [_ w409]
          tunnel: w399 -> [_ w408]
          tunnel: [w406 w407] -> w397
          frame False {
          }
          frame True {
            n124 = call-poly <vilib>:"DAQmx Write.vi"("task/channels in"=w408, "data"=w409, "error in"=w410) -> ("error out"=w407:errorcluster)  [unwired: 10 in, 2 out]
          }
        }
      }
      event "write": Value Change {
        n125 = event-data() -> ()  [unwired: 1 in, 6 out]
        n126 = Enqueue Element(queue=w421, element="load", error in (no error)=w420) -> ()  [unwired: 1 in, 3 out]
      }
      event "Normal": Value Change {
        n127 = event-data() -> ()  [unwired: 1 in, 6 out]
        n128 = local read "Output Array"() -> (w430:T1)
        n129 = local read "SampQuant.SampPerChan"() -> (w429:dbl)
        n130 = local read "square wave duty cycle (%)"() -> (w426:dbl)
        n131 = local read "SampClk.Rate"() -> (w428:dbl)
        n132 = local read "offset"() -> (w425:dbl)
        n133 = local read "DAQ Simulation"() -> (w423:bool)
        n134 = Bundle By Name(cluster=cluster{"Fs":dbl, "#s":dbl} {"Fs"=1000.0, "#s"=1000.0} ("sampling info"), "#s"=w429, "Fs"=w428) -> (w433:cluster{"Fs":dbl, "#s":dbl})
        n135 = for {
          tunnel: w433 -> [w447]
          tunnel: [w446] -> w432
          tunnel: [w445] -> w431 mode=indexing
          tunnel: w430 -> [w444] mode=indexing
          tunnel: w426 -> [w440]
          tunnel: w425 -> [w439]
          n136 = Unbundle By Name(w444) -> ("Waveform Type"=w443:u16, "Frequency"=w442:dbl, "Amplitude"=w441:dbl)
          n137 = call <vilib>:"Basic Function Generator.vi"("offset"=w439, "square wave duty cycle (%)"=w440, "sampling info"=w447, "signal type"=w443, "amplitude"=w441, "frequency"=w442) -> ("error out"=w446:errorcluster, "signal out"=w445:waveform(dbl))  [unwired: 3 in, 1 out]
        }
        n138 = case shown="True" w423 {
          tunnel: w432 -> [w434 w438]
          tunnel: w431 -> [_ w437]
          tunnel: [w434 w435] -> w424
          frame False {
          }
          frame True {
            n139 = local read "task out"() -> (w436:refnum<k21>)
            n140 = call-poly <vilib>:"DAQmx Write.vi"("task/channels in"=w436, "data"=w437, "error in"=w438) -> ("error out"=w435:errorcluster)  [unwired: 10 in, 2 out]
          }
        }
      }
      event "aquisition": Value Change {
        w448 = 10178 items=["Finite Samples"=10178, "Continuous Samples"=10123, "Hardware Timed Single Point"=12522] ("Sample Mode")
        n141 = event-data() -> ()  [unwired: 1 in, 6 out]
        n142 = Enqueue Element(queue=w455, element="daqstart", error in (no error)=w454) -> (queue out=w452:refnum<queue>, error out=w451:errorcluster)  [unwired: 1 in, 1 out]
        n143 = Enqueue Element(queue=w452, element="aquisition", error in (no error)=w451) -> (queue out=w450:refnum<queue>, error out=w449:errorcluster)  [unwired: 1 in, 1 out]
        n144 = local write "Sample Mode"(w448) -> ()
      }
      event "AO Start": Value Change {
        w457 = 10123 items=["Finite Samples"=10178, "Continuous Samples"=10123, "Hardware Timed Single Point"=12522] ("Sample Mode")
        n145 = event-data() -> ()  [unwired: 1 in, 6 out]
        n146 = Enqueue Element(queue=w461, element="daqstart", error in (no error)=w459) -> (queue out=w460:refnum<queue>, error out=w458:errorcluster)  [unwired: 1 in, 1 out]
        n147 = Enqueue Element(queue=w460, element="aostart", error in (no error)=w458) -> (queue out=w464:refnum<queue>, error out=w463:errorcluster)  [unwired: 1 in, 1 out]
        n148 = local write "Sample Mode"(w457) -> ()
      }
    }
  }
  n149 = Merge Errors(w7, w6) -> (w4:errorcluster)
  n150 = Flush Queue(queue=w5, error in (no error)=w4) -> (queue out=w3:refnum<queue>, error out=w2:errorcluster)  [unwired: 1 out]
  n151 = Release Queue(queue=w3, error in (no error)=w2) -> ()  [unwired: 1 in, 3 out]
